vi "PCO_ConvertCreate.vi"(8 "error in (no error)":errorcluster {"code" format="%x"}, 9 "iConvertType":i32(ring)=2 items=["PCO_BW_CONVERT"=1, "PCO_COLOR_CONVERT"=2, "PCO_PSEUDO_CONVERT"=3, "PCO_COLOR16_CONVERT"=4], 10 "strSensor":T1 {"iSensorInfoBits" items=["CONVERT_SENSOR_COLORIMAGE"=1, "CONVERT_SENSOR_UPPERALIGNED"=2]}) -> (0 "error out":errorcluster {"code" format="%x"}, 2 "ErrorMessage":i32 format="%x", 3 "ph out":u64)   [LabVIEW 2019, in "Convert.lvlib"]
doc: "int PCOCONVERT_API PCO_ConvertCreate(HANDLE* ph, PCO_SensorInfo *strSensor, int iConvertType);"
uses:
  Convert.lvlib
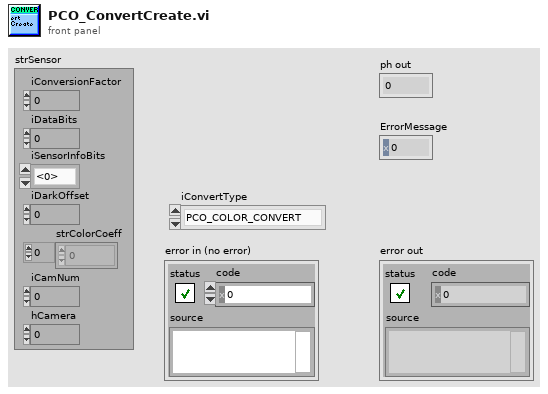
[diagram p1: front panel]
types:
  T1 = cluster{"iConversionFactor":i32, "iDataBits":i32, "iSensorInfoBits":i32, "iDarkOffset":i32, "strColorCoeff":dbl[], "iCamNum":i32, "hCamera":u64}
  T2 = cluster{"wSize":u16, "wDummy":u16, "iConversionFactor":i32, "iDataBits":i32, "iSensorInfoBits":i32, "iDarkOffset":i32, "dwzzDummy0":u32, "strColorCoeff":cluster{dbl, dbl, dbl, dbl, dbl, dbl, dbl, dbl, dbl}, "iCamNum":i32, "hCamera":u64, "dwzzDummy1":cluster{u32, u32, u32, u32, u32, u32, u32, u32, u32, u32, u32, u32, u32, u32, u32, u32, u32, u32, u32, u32, u32, u32, u32, u32, u32, u32, u32, u32, u32, u32, u32, u32, u32, u32, u32, u32, u32, u32, u32}}
  T3 = cluster{"wSize":u16, "wDummy":u16, "iConversionFactor":i32, "iDataBits":i32, "iSensorInfoBits":i32, "iDarkOffset":i32, "dwzzDummy0":u32, "strColorCoeff":cluster{dbl, dbl, dbl, dbl, dbl, dbl, dbl, dbl, dbl}, "iCamNum":i32, "hCamera":u32, "dwzzDummy1":cluster{u32, u32, u32, u32, u32, u32, u32, u32, u32, u32, u32, u32, u32, u32, u32, u32, u32, u32, u32, u32, u32, u32, u32, u32, u32, u32, u32, u32, u32, u32, u32, u32, u32, u32, u32, u32, u32, u32}}
  T4 = cluster{u32, u32, u32, u32, u32, u32, u32, u32, u32, u32, u32, u32, u32, u32, u32, u32, u32, u32, u32, u32, u32, u32, u32, u32, u32, u32, u32, u32, u32, u32, u32, u32, u32, u32, u32, u32, u32, u32, u32}
  T5 = cluster{"strColorCoeff[0]":dbl, "strColorCoeff[1]":dbl, "strColorCoeff[2]":dbl, "strColorCoeff[3]":dbl, "strColorCoeff[4]":dbl, "strColorCoeff[5]":dbl, "strColorCoeff[6]":dbl, "strColorCoeff[7]":dbl, "strColorCoeff[8]":dbl}
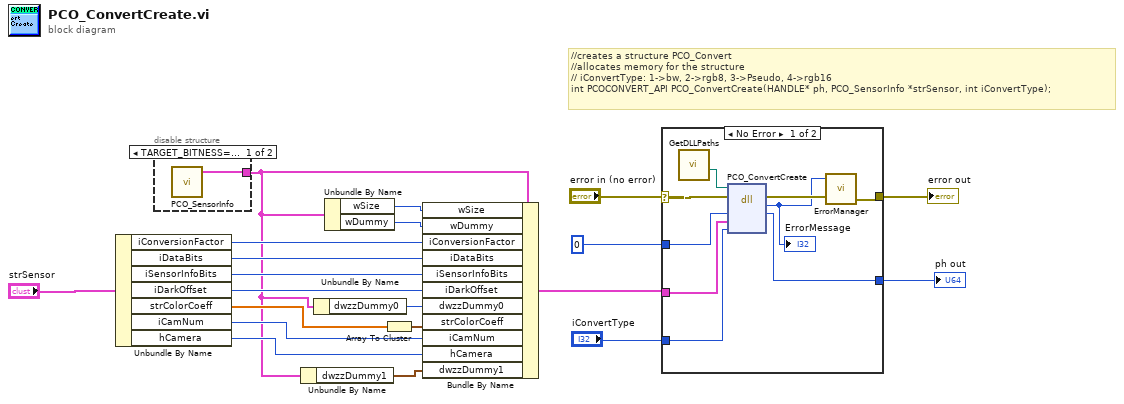
[diagram p0: block diagram]
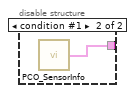
[diagram p2: hidden frame]
diagram:
  # "//creates a structure PCO_Convert\n//allocates memory for the structure\n// iConvertType: 1->bw, 2->rgb8, 3->Pseudo, 4->rgb16\nint PCOCONVERT_API PCO_ConvertCreate(HANDLE* ph, PCO_SensorInfo *strSensor, int iConvertType);"
  n1 = Unbundle By Name("strSensor") -> ("iConversionFactor"=w14:i32, "iDataBits"=w13:i32, "iSensorInfoBits"=w12:i32, "iDarkOffset"=w11:i32, "strColorCoeff"=w16:dbl[], "iCamNum"=w10:i32, "hCamera"=w9:u64)
  n2 = disable-structure "Diagram Disable Structure" shown="TARGET_BITNESS==64, Default" {
    disable-tunnel: [w21 w22] -> w4
    frame condition #0 (active) {
      n3 = call "PCO_SensorInfo.vi"() -> ("PCO_SensorInfo_Raw_x64"=w21:T2)  [unwired: 4 in, 4 out]
    }
    frame condition #1 {
      n4 = call "PCO_SensorInfo.vi"() -> ("PCO_SensorInfo_Raw_win32"=w22:T3)  [unwired: 4 in, 4 out]
    }
  }
  n5 = Unbundle By Name(w4) -> ("dwzzDummy1"=w8:T4)
  n6 = Unbundle By Name(w4) -> ("dwzzDummy0"=w7:u32)
  n7 = Unbundle By Name(w4) -> ("wSize"=w6:u16, "wDummy"=w5:u16)
  n8 = Array To Cluster(array=w16) -> (cluster=w15:T5)
  n9 = Bundle By Name(cluster=w4, "wSize"=w6, "wDummy"=w5, "iConversionFactor"=w14, "iDataBits"=w13, "iSensorInfoBits"=w12, "iDarkOffset"=w11, "dwzzDummy0"=w7, "strColorCoeff"=w15, "iCamNum"=w10, "hCamera"=w9, "dwzzDummy1"=w8) -> (w3:T2)
  n10 = case shown="No Error" "error in (no error)" {
    selector: "error in (no error)" -> [w24 w33]
    tunnel: u64 0 ("ph") -> [w31 w32]
    tunnel: [w30 w32] -> w20
    tunnel: w3 -> [w29 _]
    tunnel: "iConvertType" -> [w28 _]
    tunnel: [w26 w33] -> w19
    frame No Error {
      n11 = call "GetDLLPaths.vi"() -> ("PCO_Conv_Path"=w23:path)  [unwired: 8 in, 3 out]
      n12 = dll-call lib="?" fn="PCO_ConvertCreate"(path in=w23, error in=w24, "ph"=w31, "strSensor"=w29, "iConvertType"=w28) -> (error out=w27:errorcluster, "return type"=w25:i32, "ph"=w30:u64)  [unwired: 3 in, 1 out]
      "ErrorMessage" <- w25
      n13 = call "ErrorManager.vi"("error in (no error)"=w27, "error code"=w25) -> ("error out"=w26:errorcluster)  [unwired: 2 in, 1 out]
    }
    frame Error {
    }
  }
  "ph out" <- w20
  "error out" <- w19
